vi "Translate_COMBOBOX.vi"(8 "error IN":errorcluster, 10 "Cle":string, 11 "CmbBox Refnum":refnum<vi>) -> (0 "error out":errorcluster)   [LabVIEW 2011]
uses:
  Dictionnary/EnumCommandDictionnaire.ctl
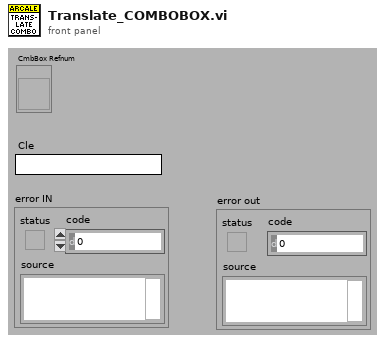
[diagram p1: front panel]
types:
  T1 = typedef "EnumCommandDictionnaire.ctl" = enum16{"Load", "Translate", "Save", "GetDico", "Set : A traduire = Vrai", "Set : A Traduire = Faux", "SetDico"}
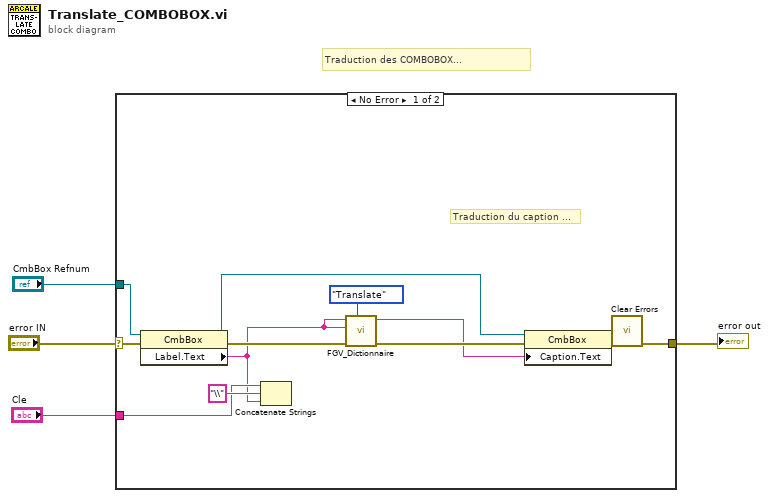
[diagram p0: block diagram]
diagram:
  # "Traduction des COMBOBOX..."
  n1 = case shown="No Error" "error IN" {
    selector: "error IN" -> [w16 w17]
    tunnel: "CmbBox Refnum" -> [w15 _]
    tunnel: "Cle" -> [w11 _]
    tunnel: [w6 w17] -> w1
    frame No Error {
      # "Traduction du caption ..."
      n2 = property class="CmbBox"(reference=w15, error in=w16) -> (reference out=w12:refnum<vi>, error out=w9:errorcluster, "Label.Text"=w5:string)
      n3 = Concatenate Strings(w11, "\\" ("string"), w5) -> ()  [unwired: 1 out]
      n4 = call "FGV_Dictionnaire.vi"("Command"=EnumCommandDictionnaire."Translate", "error in (no error)"=w9, "Chaîne"=w5, "Clé"=w5) -> ("error out"=w8:errorcluster, "Traduction"=w7:string)  [unwired: 5 in, 1 out]
      n5 = property class="CmbBox"(reference=w12, error in=w8, "Caption.Text"=w7) -> (error out=w13:errorcluster)  [unwired: 1 out]
      n6 = call <vilib>:"Clear Errors.vi"("error in (no error)"=w13) -> ("error out"=w6:errorcluster)  [unwired: 6 in]
    }
    frame Error {
    }
  }
  "error out" <- w1
